vi "RebuildAction.vi"(8 "error in (no error)":errorcluster, 11 "TrayIcon in":refnum<class "MGI_TrayIcon.lvclass">) -> (0 "error out":errorcluster, 3 "TrayIcon out":refnum<class "MGI_TrayIcon.lvclass">)   [LabVIEW 2016, in "MGI_TrayIcon.lvclass"]
doc: "Authored by Derek E. Trepanier\nsupport@mooregoodideas.com\nwww.mooregoodideas.com\n\nCopyright (c) 2012, Moore Good Ideas, Inc.\n\nAll rights reserved.\n\nRedistribution and use in source and binary forms, with or without modification, are permitted provided that the following conditions are met:\n\n * Redistributions of source code must retain the above copyright notice, this list of conditions and the following disclaimer.\n * Redistributions in binary form must reproduce the above copyright notice, this list of conditions and the following disclaimer in the documentation and/or other materials provided with the distribution.\n * Neither the name of Moore Good Ideas, Inc. nor the names of its contributors may be used to endorse or promote products derived from this software without specific prior written permission.\n\nTHIS SOFTWARE IS PROVIDED BY THE COPYRIGHT HOLDERS AND CONTRIBUTORS \"AS IS\" AND ANY EXPRESS OR IMPLIED WARRANTIES, INCLUDING, BUT NOT LIMITED TO, THE IMPLIED WARRANTIES OF MERCHANTABILITY AND FITNESS FOR A PARTICULAR PURPOSE ARE DISCLAIMED. IN NO EVENT SHALL THE COPYRIGHT OWNER OR CONTRIBUTORS BE LIABLE FOR ANY DIRECT, INDIRECT, INCIDENTAL, SPECIAL, EXEMPLARY, OR CONSEQUENTIAL DAMAGES (INCLUDING, BUT NOT LIMITED TO, PROCUREMENT OF SUBSTITUTE GOODS OR SERVICES; LOSS OF USE, DATA, OR PROFITS; OR BUSINESS INTERRUPTION) HOWEVER CAUSED AND ON ANY THEORY OF LIABILITY, WHETHER IN CONTRACT, STRICT LIABILITY, OR TORT (INCLUDING NEGLIGENCE OR OTHERWISE) ARISING IN ANY WAY OUT OF THE USE OF THIS SOFTWARE, EVEN IF ADVISED OF THE POSSIBILITY OF SUCH DAMAGE."
uses:
  <userlib>/_MGI/Menu Building/MenuTypes/TrayIcon/MGI_TrayIcon.lvclass
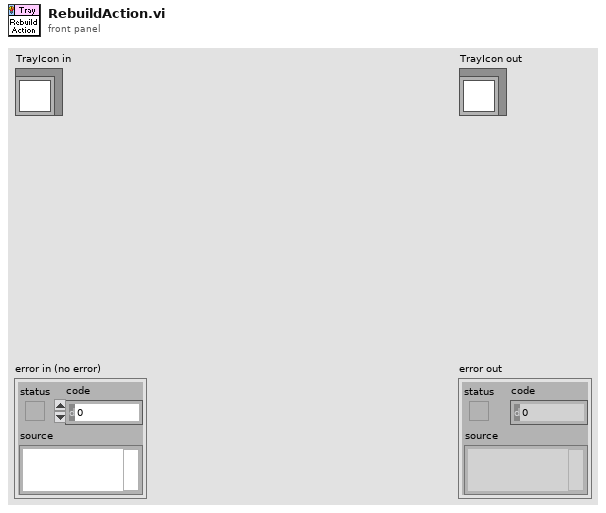
[diagram p1: front panel]
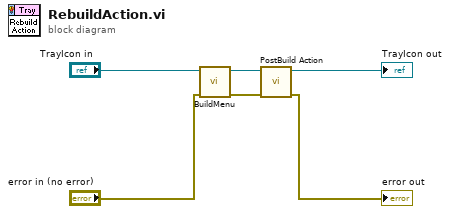
[diagram p0: block diagram]
diagram:
  n1 = call-dynamic "BuildMenu.vi"("error in (no error)"="error in (no error)", "Menu in"="TrayIcon in") -> ("error out"=w2:errorcluster, "Menu out"=w6:refnum<class "MGI_TrayIcon.lvclass">)  [unwired: 8 in]
  n2 = call-dynamic "PostBuild Action.vi"("error in (no error)"=w2, "MGI_TrayIcon in"=w6) -> ("error out"=→"error out":errorcluster, "MGI_TrayIcon out"=→"TrayIcon out":refnum<class "MGI_TrayIcon.lvclass">)  [unwired: 8 in]
